vi "Read Digital DAQ.vi"(8 "error in (no error)":errorcluster, 10 "Digital Inputs":bool[](array[boolean]), 11 "User Interface in":refnum<class "User Interface.lvclass">) -> (0 "error out":errorcluster, 3 "User Interface out":refnum<class "User Interface.lvclass">)   [LabVIEW 2015, in "User Interface.lvlib" / "User Interface.lvclass"]
uses:
  User Interface.lvclass
  Controls/Car Wash Indicators.ctl
  User Interface.lvclass/User Interface.ctl
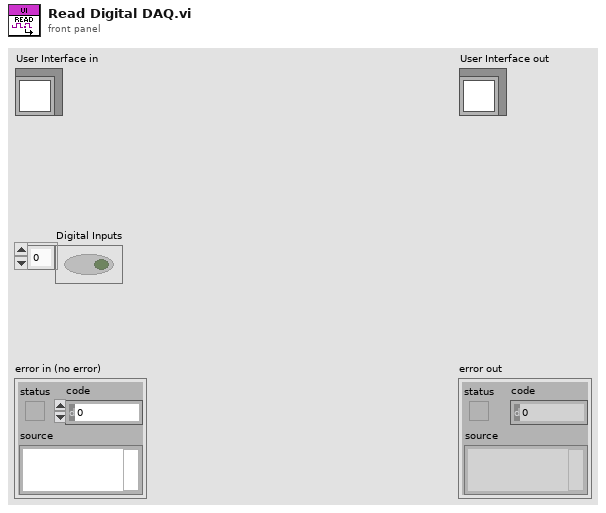
[diagram p1: front panel]
types:
  T1 = typedef "Car Wash Indicators.ctl" = cluster{"Soapy Water":bool, "High Pressure Wash":bool, "Air Dry":bool, "Vehicle Out of Position":bool}
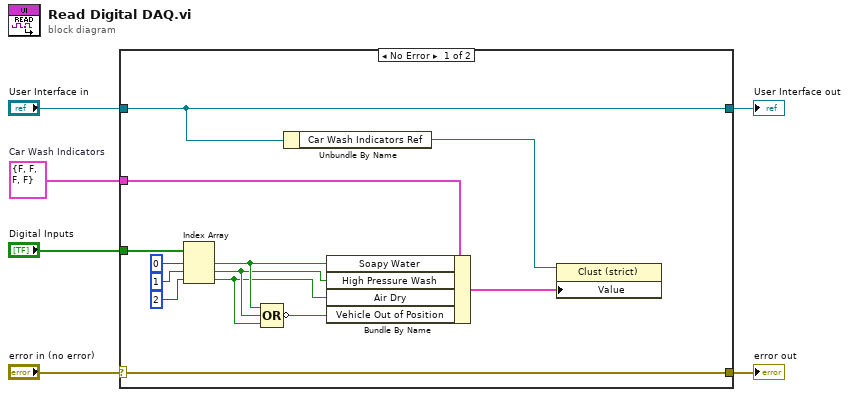
[diagram p0: block diagram]
diagram:
  w2 = T1 {"Soapy Water"=FALSE, "High Pressure Wash"=FALSE, "Air Dry"=FALSE, "Vehicle Out of Position"=FALSE}  # Car Wash Indicators
  n1 = case shown="No Error" "error in (no error)" {
    selector: "error in (no error)" -> [w19 w21]
    tunnel: [w19 w21] -> w5
    tunnel: [w9 w20] -> w3
    tunnel: "User Interface in" -> [w9 w20]
    tunnel: w2 -> [w18 _]
    tunnel: "Digital Inputs" -> [w17 _]
    frame No Error {
      n2 = Index Array(array=w17, index #1=0 ("index"), index #2=1 ("index"), index #3=2 ("index")) -> (element #1=w13:bool, element #2=w12:bool, element #3=w11:bool)
      n3 = Compound Arithmetic op=OR(w13, w12, w11) -> (invert w10:bool)
      n4 = Unbundle By Name(w9) -> ("Car Wash Indicators Ref"=w8:refnum<vi>)
      n5 = Bundle By Name(cluster=w18, "Soapy Water"=w13, "High Pressure Wash"=w12, "Air Dry"=w11, "Vehicle Out of Position"=w10) -> (w7:T1)
      n6 = property class="Clust (strict)"(reference=w8, "Value"=w7) -> ()  [unwired: 1 in, 2 out]
    }
    frame Error {
    }
  }
  "error out" <- w5
  "User Interface out" <- w3
